vi "Telnet Connection Destructor.vi"(0 "object data in":T1) -> ()   [LabVIEW 2015]
doc: "Function that cleans up when an object is destroyed.\nIt may close a file or connection, or may need to trigger an occurrence."
uses:
  Telnet Connection Data.ctl
  Semaphore RefNum.ctl
panel:
  out "error out":errorcluster
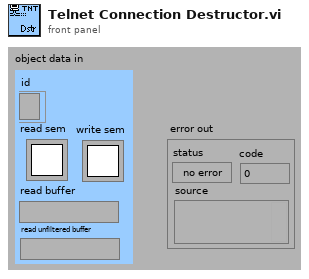
[diagram p1: front panel]
types:
  T1 = typedef "Telnet Connection Data.ctl" = cluster{"id":refnum<k5>, "read sem":T2, "write sem":T2, "read buffer":string, "read unfiltered buffer":string}
  T2 = typedef "Semaphore RefNum.ctl" = refnum<k1>
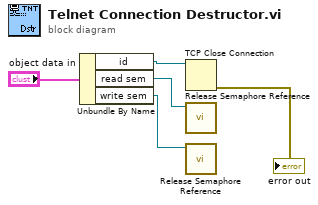
[diagram p0: block diagram]
diagram:
  n1 = Unbundle By Name("object data in") -> ("id"=w4:refnum<k5>, "read sem"=w3:T2, "write sem"=w2:T2)
  n2 = TCP Close Connection(connection ID=w4) -> (error out=→"error out":errorcluster)  [unwired: 2 in, 1 out]
  n3 = call <vilib>:"Release Semaphore Reference.vi"("semaphore"=w3) -> ()  [unwired: 9 in, 2 out]
  n4 = call <vilib>:"Release Semaphore Reference.vi"("semaphore"=w2) -> ()  [unwired: 9 in, 2 out]
